vi "Global.vi"() -> ()   [LabVIEW 2017, in "nifxpmath_Sqrt.xnode"]
uses:
  <vilib>/rvi/FXPMathLib/FxpSqrt/XNode/nifxpmath_Sqrt.xnode
panel:
  out "SMALL ICON w/ 4WIRE":picture
  in  "SMALL ICON":picture
  out "NORMAL BANNER":picture
  in  "TERM SQRT NAME":string="sqrt(x)"
  in  "TERM X NAME":string="x"
  in  "TERM X ID":string="TERM_X"
  in  "TERM SQRT ID":string="TERM_SQRT"
  in  "TERM OVERFLOW ID":string="TERM_OVFL"
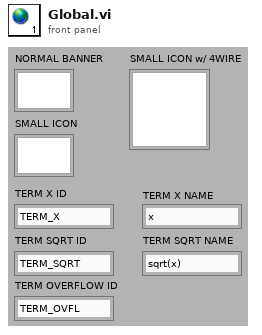
[diagram p1: front panel]
diagram:
